vi "Label.vi"(8 "error in (no error)":errorcluster, 11 "Node Ptr":T1 format="%.0x") -> (0 "error out":errorcluster)   [LabVIEW 2020, in "Ballard ARINC 429 System Explorer.lvlib" / "Implementation.lvlib"]
uses:
  Implementation.lvlib
  <vilib>/NI VeriStand/Custom Device API/Custom Device API.lvlib
  Scripting/Ballard ARINC 429 Scripting.lvlib
  <vilib>/NI VeriStand/Custom Device API/Custom Device Item Ref.ctl
panel:
  out "SDI Enabled":bool
  out "SDI":u8
  out "Label (octal)":i32 format="%o"
  out "Label (decimal)":i32
  in  "SHDocVw.IWebBrowser":refnum<k7>(container)
  in  "General Header":cluster{"Section Name":string}={"Section Name"="Ballard ARINC 429 - Label"}
  in  "Description":string
  out "Name":string
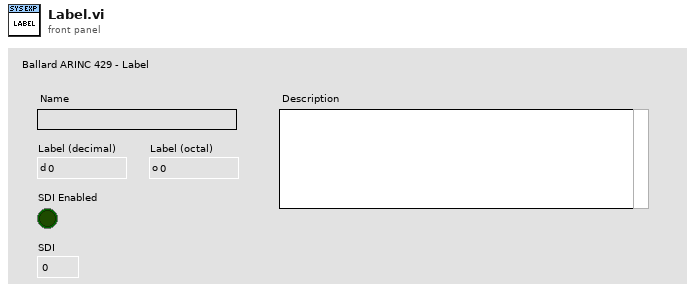
[diagram p1: front panel]
types:
  T1 = typedef "Custom Device API.lvlib/Custom Device Item Ref.ctl" = u64
  T2 = typedef "Custom Device API.lvlib/Custom Device Item Info.ctl" = cluster{"Name":string, "Is Channel":bool, "GUID":string, "Is Waveform":bool}
  T3 = typedef "Label Properties.ctl" = cluster{"label (Dec)":i32, "SDI value":u8, "SDI enabled":bool}
  T4 = typedef "Custom Device API.lvlib/Custom Device Commands.ctl" = enum16{"Default", "Item renamed", "Shutdown", "Dynamic button pressed"}
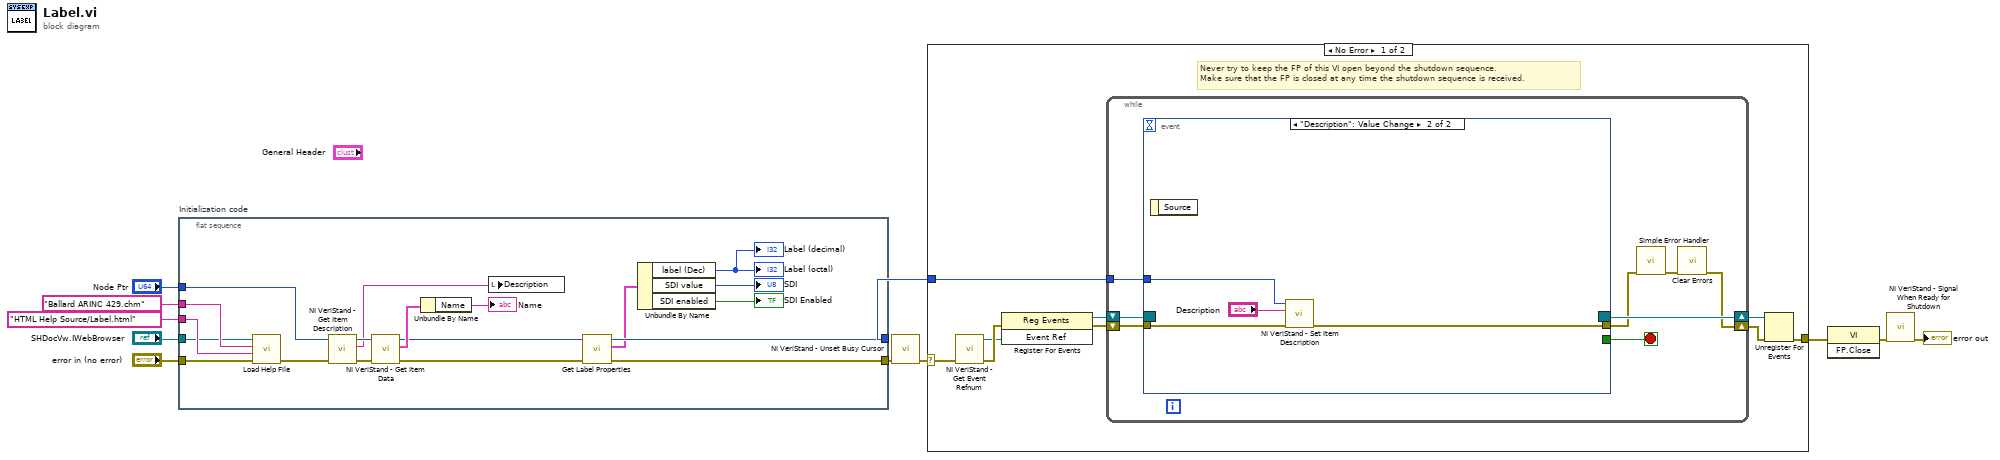
[diagram p0: block diagram]
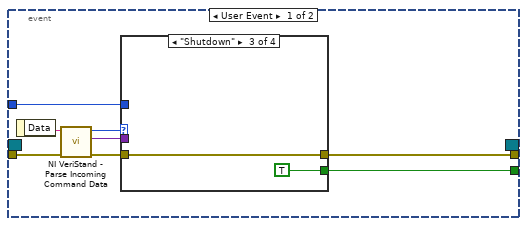
[diagram p2: hidden frame]
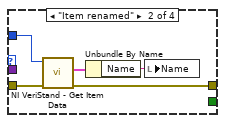
[diagram p4: hidden frame]
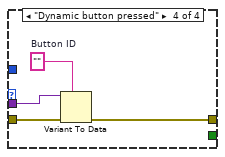
[diagram p5: hidden frame]
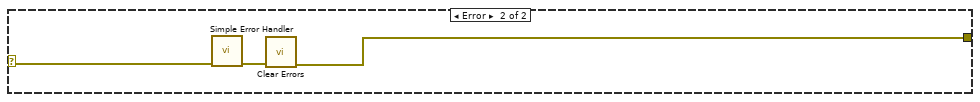
[diagram p6: hidden frame]
diagram:
  n1 = flat-sequence "Initialization code" {
    tunnel: "error in (no error)" -> [w25]
    tunnel: "Node Ptr" -> [w27]
    tunnel: [w16] -> w7
    tunnel: [w18] -> w4
    tunnel: "SHDocVw.IWebBrowser" -> [w21]
    tunnel: "HTML Help Source/Label.html" ("CD_CHM_Section") -> [w23]
    tunnel: "Ballard ARINC 429.chm" ("CD_CHM_FileName") -> [w22]
    frame #0 {
      n2 = call "Load Help File.vi"("error in (no error)"=w25, "HTML File to Load"=w23, "Main CHM File"=w22, "Browser"=w21) -> ("error out"=w24:errorcluster)  [unwired: 7 in]
      n3 = call <vilib>:"NI VeriStand - Get Item Description.vi"("error in (no error)"=w24, "Item Ref in"=w27) -> ("error out"=w29:errorcluster, "Description"=w26:string, "Item Ref out"=w30:T1)  [unwired: 7 out]
      n4 = call <vilib>:"NI VeriStand - Get Item Data.vi"("error in (no error)"=w29, "Item Ref in"=w30) -> ("error out"=w17:errorcluster, "Item Info"=w28:T2, "Item Ref out"=w19:T1)  [unwired: 7 out]
      n5 = Unbundle By Name(w28) -> ("Name"=→"Name":string)
      n6 = local write "Description"(w26) -> ()
      n7 = call "Get Label Properties.vi"("error in"=w17, "label ref in"=w19) -> ("error out"=w16:errorcluster, "label properties"=w15:T3, "label ref out"=w18:T1)  [unwired: 7 in]
      n8 = Unbundle By Name(w15) -> ("label (Dec)"=→"Label (decimal)" →"Label (octal)":i32, "SDI value"=→"SDI":u8, "SDI enabled"=→"SDI Enabled":bool)
    }
  }
  n9 = call <vilib>:"NI VeriStand - Unset Busy Cursor.vi"("error in (no error)"=w7) -> ("error out"=w6:errorcluster)  [unwired: 10 out]
  n10 = case shown="No Error" w6 {
    selector: w6 -> [w31 w74]
    tunnel: [w36 w72] -> w11
    tunnel: w4 -> [w32 _]
    frame No Error {
      # "Never try to keep the FP of this VI open beyond the shutdown sequence.\nMake sure that the FP is closed at any time the shutdown sequence is received."
      n11 = call <vilib>:"NI VeriStand - Get Event Refnum.vi"("error in (no error)"=w31) -> ("error out"=w39:errorcluster, "Event Ref"=w35:refnum<user-event>)  [unwired: 9 out]
      n12 = register-events(error in=w39, w35) -> (reference out=w33:refnum<event-registration>, error out=w34:errorcluster)  [unwired: 1 in]
      n13 = while {
        tunnel: w32 -> [w43]
        shift-right: [w40] -> w37
        shift-left: w34 -> [w46]
        shift-right: [w47] -> w38
        shift-left: w33 -> [w45]
        stop <- w44 stop-if-true
        n14 = event shown="[1] \"Description\": Value Change" {
          selector: w45 -> [_ _]
          dyn-events: [_ _] -> w47
          timeout: _ -> [_ _]
          tunnel: w46 -> [w55 w70]
          tunnel: [w51 _] -> w44
          tunnel: [w50 w69] -> w42
          tunnel: w43 -> [w49 w71]
          event User Event {
            n15 = event-data() -> ("Data"=w54:string)  [unwired: 1 out]
            n16 = call <vilib>:"NI VeriStand - Parse Incoming Command Data.vi"("error in (no error)"=w55, "Incoming data"=w54) -> ("error out"=w53:errorcluster, "Outgoing data"=w48:variant, "Action"=w52:T4)  [unwired: 7 out]
            n17 = case shown="\"Shutdown\"" w52 {
              tunnel: w53 -> [w56 w61 w62 w67]
              tunnel: [_ _ TRUE _] -> w51
              tunnel: [w56 w58 w62 w64] -> w50
              tunnel: w49 -> [_ w60 _ _]
              tunnel: w48 -> [_ _ _ w66]
              frame "Default", Default {
              }
              frame "Item renamed" {
                n18 = call <vilib>:"NI VeriStand - Get Item Data.vi"("error in (no error)"=w61, "Item Ref in"=w60) -> ("error out"=w58:errorcluster, "Item Info"=w59:T2)  [unwired: 8 out]
                n19 = Unbundle By Name(w59) -> ("Name"=w57:string)
                n20 = local write "Name"(w57) -> ()
              }
              frame "Shutdown" {
              }
              frame "Dynamic button pressed" {
                w65 = ""  # Button ID
                n21 = Variant To Data(error in=w67, type=w65, Variant=w66) -> (error out=w64:errorcluster)  [unwired: 1 out]
              }
            }
          }
          event "Description": Value Change {
            n22 = event-data() -> ()  [unwired: 2 out]
            n23 = call <vilib>:"NI VeriStand - Set Item Description.vi"("error in (no error)"=w70, "Description"="Description", "Item Ref in"=w71) -> ("error out"=w69:errorcluster)  [unwired: 8 out]
          }
        }
        n24 = call <vilib>:"Simple Error Handler.vi"("error in (no error)"=w42) -> ("error out"=w41:errorcluster)  [unwired: 1 in, 7 out]
        n25 = call <vilib>:"Clear Errors.vi"("error in (no error)"=w41) -> ("error out"=w40:errorcluster)  [unwired: 1 in, 5 out]
      }
      n26 = Unregister For Events(event registration refnum=w38, error in=w37) -> (error out=w36:errorcluster)
    }
    frame Error {
      n27 = call <vilib>:"Simple Error Handler.vi"("error in (no error)"=w74) -> ("error out"=w73:errorcluster)  [unwired: 1 in, 7 out]
      n28 = call <vilib>:"Clear Errors.vi"("error in (no error)"=w73) -> ("error out"=w72:errorcluster)  [unwired: 1 in, 5 out]
    }
  }
  n29 = invoke class="VI" method="FP.Close"(error in=w11) -> (error out=w10:errorcluster)  [unwired: 2 in, 2 out]
  n30 = call <vilib>:"NI VeriStand - Signal When Ready for Shutdown.vi"("error in (no error)"=w10) -> ("error out"=→"error out":errorcluster)  [unwired: 10 out]
